vi "test Add Find Remove Alias.vi"(8 "error in (no error)":errorcluster, 11 "TestCase in":refnum<class "Routing and Faulting Scripting Unit Tests.lvclass">) -> (0 "error out":errorcluster, 3 "TestCase out":refnum<class "Routing and Faulting Scripting Unit Tests.lvclass">)   [LabVIEW 2017, in "Routing and Faulting Scripting Unit Tests.lvclass"]
uses:
  Routing and Faulting Scripting Unit Tests.lvclass
  Shared/Alias Mapping.ctl
  Shared/Alias Endpoint.ctl
  Routing and Faulting Scripting Unit Tests.lvclass/Routing and Faulting Scripting Unit Tests.ctl
  <vilib>/addons/_JKI Toolkits/VI Tester/TestCase.llb/TestCase.lvclass
  Routing and Faulting Scripting.lvlib
  Shared/Routing and Faulting Shared.lvlib
  C:/Program Files (x86)/National Instruments/LabVIEW 2017/vi.lib/addons/_JKI Toolkits/VI Tester/TestCase.llb/TestCase.lvclass
panel:
  in  "Save?":bool
  out "Output Filename":string
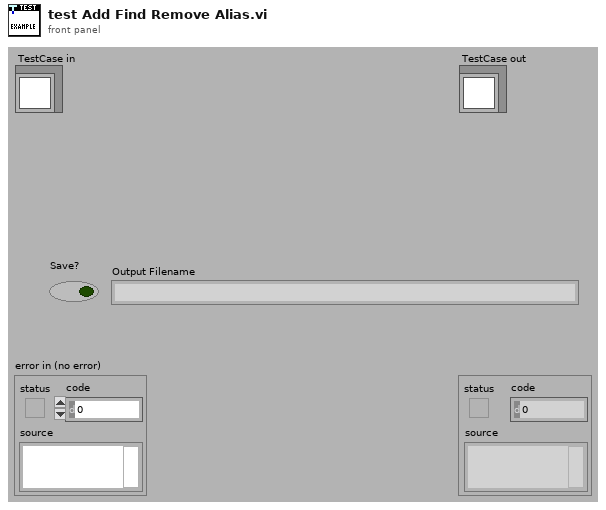
[diagram p1: front panel]
types:
  T1 = typedef "Routing and Faulting Shared.lvlib/Alias Endpoint.ctl" = cluster{"Module Path":string, "Endpoint":string}
  T2 = typedef "Routing and Faulting Shared.lvlib/Alias Mapping.ctl" = cluster{"Alias":string, "Endpoint":T1}
  T3 = typedef "Custom Device API.lvlib/Custom Device Item Ref.ctl" = u64
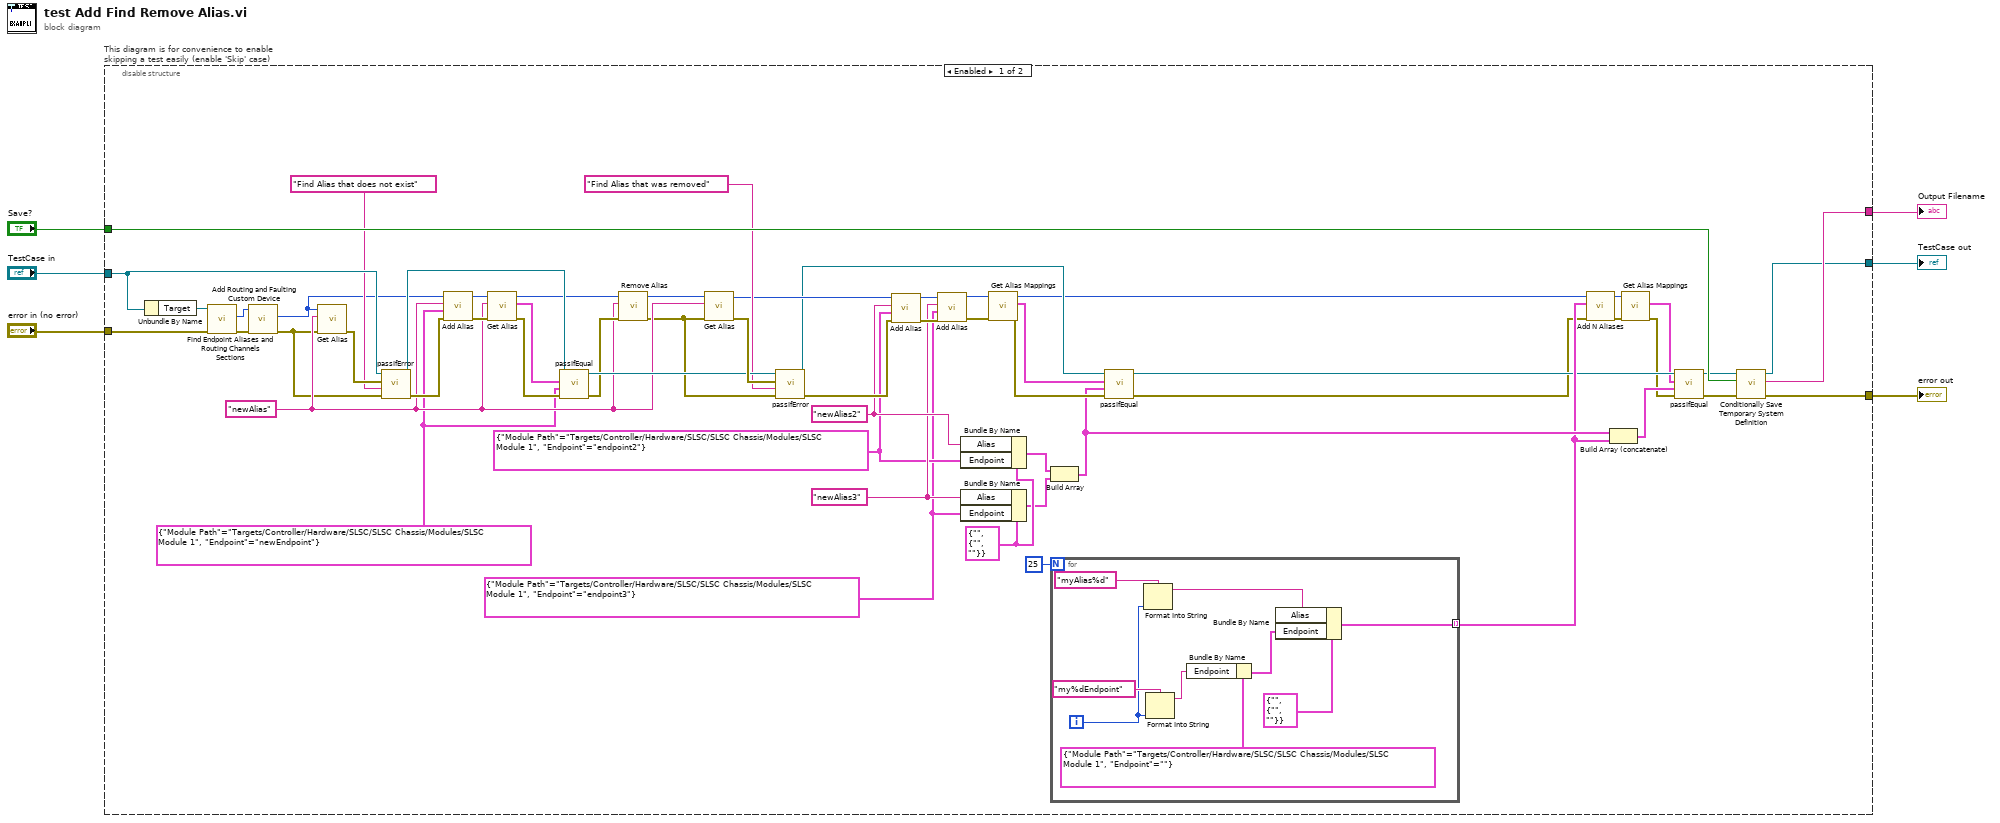
[diagram p0: block diagram]
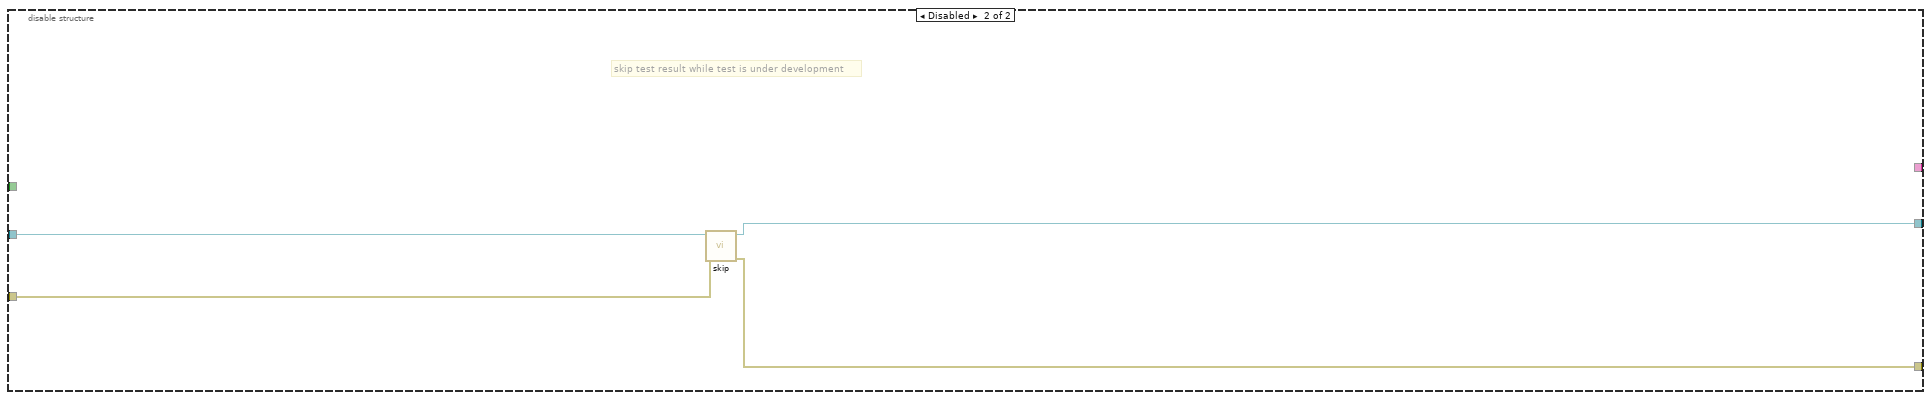
[diagram p2: hidden frame]
diagram:
  n1 = disable-structure "This diagram is for convenience to enable skipping a test easily (enable 'Skip' case)" shown="Enabled" {
    disable-tunnel: "TestCase in" -> [w57 w76]
    disable-tunnel: [w61 w74] -> w3
    disable-tunnel: [w62 w75] -> w5
    disable-tunnel: "error in (no error)" -> [w59 w73]
    disable-tunnel: [w63 _] -> w2
    disable-tunnel: "Save?" -> [w58 _]
    frame Enabled {
      w7 = T1 {"Module Path"="Targets/Controller/Hardware/SLSC/SLSC Chassis/Modules/SLSC Module 1", "Endpoint"="endpoint3"} ("Endpoint")
      w8 = T1 {"Module Path"="Targets/Controller/Hardware/SLSC/SLSC Chassis/Modules/SLSC Module 1", "Endpoint"="endpoint2"} ("Endpoint")
      w9 = T1 {"Module Path"="Targets/Controller/Hardware/SLSC/SLSC Chassis/Modules/SLSC Module 1", "Endpoint"="newEndpoint"} ("Endpoint")
      w28 = T2 {"Alias"="", "Endpoint"={"Module Path"="", "Endpoint"=""}} ("Alias Mapping")
      w29 = "newAlias3" ("Alias")
      w30 = "newAlias2" ("Alias")
      w41 = "newAlias" ("Alias")
      n2 = Unbundle By Name(w57) -> ("Target"=w60:refnum<k24>)
      n3 = call "Add Routing and Faulting Custom Device.vi"("error in (no error)"=w59, "Target in"=w60) -> ("error out"=w54:errorcluster, "Routing and Faulting Custom Device Ref"=w24:T3)  [unwired: 7 in, 1 out]
      n4 = call "Find Endpoint Aliases and Routing Channels Sections.vi"("error in (no error)"=w54, "Routing and Faulting Custom Device Ref in"=w24) -> ("error out"=w25:errorcluster, "Endpoint Aliases Ref"=w23:T3)  [unwired: 6 in, 2 out]
      n5 = call "Get Alias.vi"("error in (no error)"=w25, "Alias"=w41, "Endpoint Aliases Ref in"=w23) -> ("error out"=w56:errorcluster)  [unwired: 6 in, 2 out]
      n6 = call-dynamic "passIfError.vi"("error in (no error)"=w25, "task (\"\")"="Find Alias that does not exist" ("message (\"\")"), "error"=w56, "TestCase in"=w57) -> ("error out"=w53:errorcluster, "TestCase out"=w51:refnum<class "Routing and Faulting Scripting Unit Tests.lvclass">)  [unwired: 6 in]
      n7 = call "Add Alias.vi"("error in (no error)"=w53, "Endpoint"=w9, "Alias"=w41, "Endpoint Aliases Ref in"=w23) -> ("error out"=w48:errorcluster, "Endpoint Aliases Ref out"=w52:T3)  [unwired: 6 in]
      n8 = call "Get Alias.vi"("error in (no error)"=w48, "Alias"=w41, "Endpoint Aliases Ref in"=w52) -> ("error out"=w49:errorcluster, "Endpoint"=w50:T1, "Endpoint Aliases Ref out"=w47:T3)  [unwired: 6 in]
      n9 = call-dynamic "passIfEqual.vi"("error in (no error)"=w49, "y"=w9, "x"=w50, "TestCase in"=w51) -> ("error out"=w43:errorcluster, "TestCase out"=w45:refnum<class "Routing and Faulting Scripting Unit Tests.lvclass">)  [unwired: 6 in]
      n10 = call "Remove Alias.vi"("error in (no error)"=w43, "Alias"=w41, "Endpoint Aliases Ref in"=w47) -> ("error out"=w31:errorcluster, "Endpoint Aliases Ref out"=w44:T3)  [unwired: 7 in]
      n11 = call "Get Alias.vi"("error in (no error)"=w31, "Alias"=w41, "Endpoint Aliases Ref in"=w44) -> ("error out"=w46:errorcluster, "Endpoint Aliases Ref out"=w40:T3)  [unwired: 6 in, 1 out]
      n12 = call-dynamic "passIfError.vi"("error in (no error)"=w31, "task (\"\")"="Find Alias that was removed" ("message (\"\")"), "error"=w46, "TestCase in"=w45) -> ("error out"=w39:errorcluster, "TestCase out"=w34:refnum<class "Routing and Faulting Scripting Unit Tests.lvclass">)  [unwired: 6 in]
      n13 = call "Add Alias.vi"("error in (no error)"=w39, "Endpoint"=w8, "Alias"=w30, "Endpoint Aliases Ref in"=w40) -> ("error out"=w38:errorcluster, "Endpoint Aliases Ref out"=w37:T3)  [unwired: 6 in]
      n14 = call "Add Alias.vi"("error in (no error)"=w38, "Endpoint"=w7, "Alias"=w29, "Endpoint Aliases Ref in"=w37) -> ("error out"=w35:errorcluster, "Endpoint Aliases Ref out"=w36:T3)  [unwired: 6 in]
      n15 = Bundle By Name(cluster=w28, "Alias"=w30, "Endpoint"=w8) -> (w27:T2)
      n16 = Bundle By Name(cluster=w28, "Alias"=w29, "Endpoint"=w7) -> (w26:T2)
      n17 = call "Get Alias Mappings.vi"("error in (no error)"=w35, "Endpoint Aliases Ref in"=w36) -> ("error out"=w32:errorcluster, "Alias Mappings"=w33:T2[], "Endpoint Aliases Ref out"=w22:T3)  [unwired: 7 in]
      n18 = Build Array(w27, w26) -> (w21:T2[])
      n19 = for {
        N: 25 -> [_]
        tunnel: [w67] -> w20 mode=indexing
        i -> [w70]
        n20 = Format Into String(format string="myAlias%d" ("Alias"), w70) -> (resulting string=w68:string)  [unwired: 2 in, 1 out]
        n21 = Format Into String(format string="my%dEndpoint" ("Alias"), w70) -> (resulting string=w65:string)  [unwired: 2 in, 1 out]
        n22 = Bundle By Name(cluster=T1 {"Module Path"="Targets/Controller/Hardware/SLSC/SLSC Chassis/Modules/SLSC Module 1", "Endpoint"=""} ("Endpoint"), "Endpoint"=w65) -> (w64:T1)
        n23 = Bundle By Name(cluster=T2 {"Alias"="", "Endpoint"={"Module Path"="", "Endpoint"=""}} ("Alias Mapping"), "Alias"=w68, "Endpoint"=w64) -> (w67:T2)
      }
      n24 = call-dynamic "passIfEqual.vi"("error in (no error)"=w32, "y"=w21, "x"=w33, "TestCase in"=w34) -> ("error out"=w14:errorcluster, "TestCase out"=w16:refnum<class "Routing and Faulting Scripting Unit Tests.lvclass">)  [unwired: 6 in]
      n25 = call "Add N Aliases.vi"("error in (no error)"=w14, "Alias Mappings"=w20, "Endpoint Aliases Ref in"=w22) -> ("error out"=w18:errorcluster, "Endpoint Aliases Ref out"=w17:T3)  [unwired: 7 in]
      n26 = Build Array (concatenate)(w21, w20) -> (w19:T2[])
      n27 = call "Get Alias Mappings.vi"("error in (no error)"=w18, "Endpoint Aliases Ref in"=w17) -> ("error out"=w12:errorcluster, "Alias Mappings"=w11:T2[])  [unwired: 7 in, 1 out]
      n28 = call-dynamic "passIfEqual.vi"("error in (no error)"=w12, "y"=w19, "x"=w11, "TestCase in"=w16) -> ("error out"=w13:errorcluster, "TestCase out"=w15:refnum<class "Routing and Faulting Scripting Unit Tests.lvclass">)  [unwired: 6 in]
      n29 = call "Conditionally Save Temporary System Definition.vi"("error in (no error)"=w13, "Save?"=w58, "Test Case"=w15) -> ("error out"=w62:errorcluster, "filename"=w63:string, "Test Case"=w61:refnum<class "Routing and Faulting Scripting Unit Tests.lvclass">)  [unwired: 6 in]
    }
    frame Disabled {
      # "skip test result while test is under development"
      n30 = call <vilib>:"skip.vi"("error in (no error)"=w73, "TestCase in"=w76) -> ("error out"=w75:errorcluster, "TestCase out"=w74:refnum<class "Routing and Faulting Scripting Unit Tests.lvclass">)  [unwired: 8 in]
    }
  }
  "error out" <- w5
  "TestCase out" <- w3
  "Output Filename" <- w2
